vi "WMP.vi"() -> ()   [LabVIEW 2014]
panel:
  in  "WindowsMediaPlayer":refnum<k7>(container)
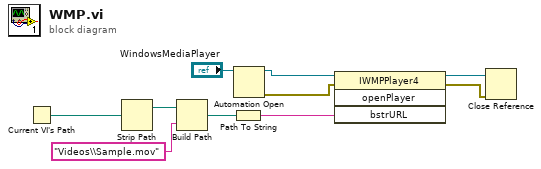
[diagram p0: block diagram]
diagram:
  n1 = Current VI's Path() -> (path=w9:path)
  n2 = Strip Path(path=w9) -> (stripped path=w8:path)  [unwired: 1 out]
  n3 = Build Path(base path=w8, name or relative path="Videos\\Sample.mov") -> (appended path=w6:path)
  n4 = Path To String(path=w6) -> (string=w5:string)
  n5 = Automation Open(Automation Refnum="WindowsMediaPlayer") -> (Automation Refnum=w3:refnum<k7>, error out=w4:errorcluster)  [unwired: 1 in, 2 out]
  n6 = invoke class="IWMPPlayer4" method="openPlayer"(reference=w3, error in=w4, "bstrURL"=w5) -> (reference out=w1:refnum<k7>, error out=w2:errorcluster)  [unwired: 1 in, 2 out]
  n7 = Close Reference(reference=w1, error in (no error)=w2) -> ()  [unwired: 1 out]
